vi "Send Command.vi"(8 "error in (no error)":errorcluster, 10 "write buffer":string, 11 "VISA resource name":refnum<visa-resource-name>) -> (0 "error out":errorcluster, 3 "VISA resource name out":refnum<visa-resource-name>)   [LabVIEW 2017]
uses:
  Microwave/Agilent PSG MXG Series/Agilent PSG MXG Series.lvlib
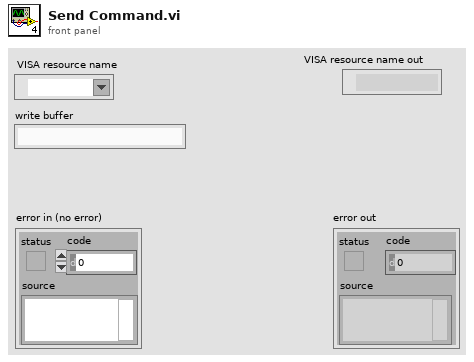
[diagram p1: front panel]
types:
  T1 = typedef "Semaphore RefNum" = refnum<k1>
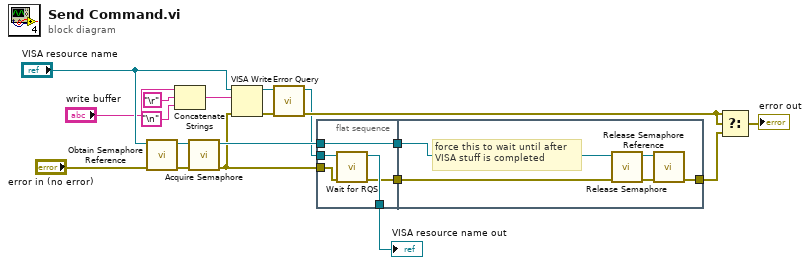
[diagram p0: block diagram]
diagram:
  n1 = call <vilib>:"Obtain Semaphore Reference.vi"("error in (no error)"="error in (no error)", "name (unnamed)"="VISA resource name") -> ("error out"=w18:errorcluster, "semaphore"=w19:T1)  [unwired: 1 in, 3 out]
  n2 = Concatenate Strings("write buffer", "\r", "\n") -> (w1:string)
  n3 = call <vilib>:"Acquire Semaphore.vi"("error in (no error)"=w18, "semaphore"=w19) -> ("error out"=w11:errorcluster, "semaphore out"=w16:T1)  [unwired: 1 in, 3 out]
  n4 = VISA Write(VISA resource name="VISA resource name", write buffer=w1, error in (no error)=w11) -> (VISA resource name out=w13:refnum<visa-resource-name>, error out=w14:errorcluster)  [unwired: 1 out]
  n5 = call "Error Query.vi"("error in (no error)"=w14, "VISA resource name"=w13) -> ("error out"=w12:errorcluster, "VISA resource name out"=w6:refnum<visa-resource-name>)  [unwired: 8 out]
  n6 = flat-sequence {
    tunnel: w11 -> [w21]
    tunnel: w16 -> [w24]
    tunnel: [w24] -> w8
    tunnel: [w20] -> w7
    tunnel: w6 -> [w23]
    tunnel: [w22] -> w5
    tunnel: [w26] -> w10
    tunnel: w8 -> [w29]
    tunnel: w7 -> [w25]
    frame #0 {
      n7 = call <vilib>:"Wait for RQS.vi"("error in (no error)"=w21, "VISA resource name"=w23) -> ("error out"=w20:errorcluster, "VISA resource name out"=w22:refnum<visa-resource-name>)  [unwired: 7 in, 1 out]
    }
    frame #1 {
      # "force this to wait until after \nVISA stuff is completed"
      n8 = call <vilib>:"Release Semaphore.vi"("error in (no error)"=w25, "semaphore"=w29) -> ("error out"=w27:errorcluster, "semaphore out"=w28:T1)  [unwired: 4 out]
      n9 = call <vilib>:"Release Semaphore Reference.vi"("error in (no error)"=w27, "semaphore"=w28) -> ("error out"=w26:errorcluster)  [unwired: 9 out]
    }
  }
  n10 = Select(t=w12, s=w12, f=w10) -> (s? t:f=→"error out":errorcluster)
  "VISA resource name out" <- w5
